vi "Read status lines.vi"(11 "httpResponse in":refnum<class "httpResponse.lvclass">) -> (1 "status chain":string[](array[string]), 2 "status":string, 3 "httpResponse out":refnum<class "httpResponse.lvclass">)   [LabVIEW 2020, in "httpClient.lvlib" / "httpResponse.lvclass"]
uses:
  httpResponse.lvclass
  httpResponse.lvclass/httpResponse.ctl
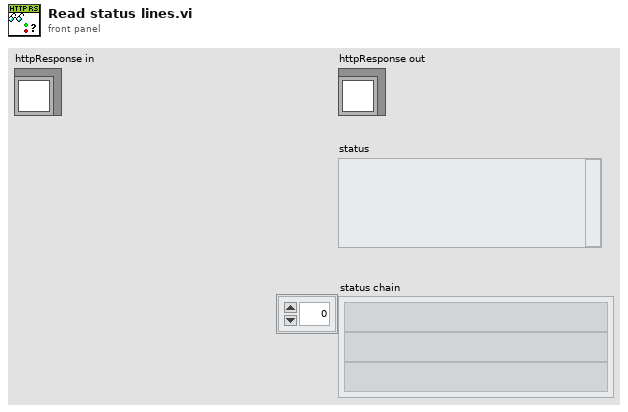
[diagram p1: front panel]
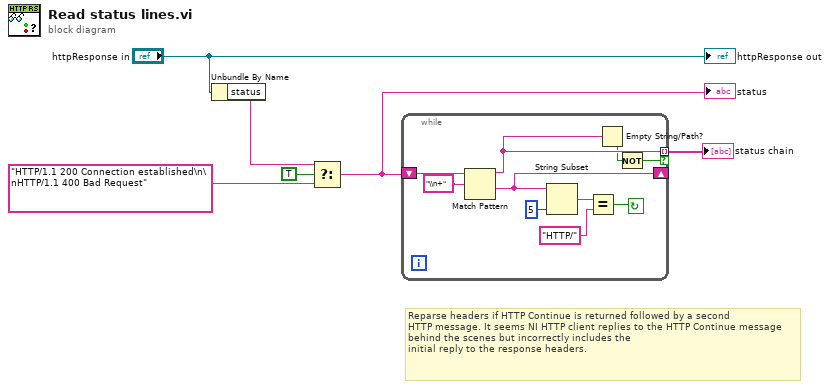
[diagram p0: block diagram]
diagram:
  # "Reparse headers if HTTP Continue is returned followed by a second\nHTTP message. It seems NI HTTP client replies to the HTTP Continue message behind the scenes but incorrectly includes the\ninitial reply to the response headers."
  n1 = Unbundle By Name("httpResponse in") -> ("status"=w2:string)
  n2 = Select(t=w2, s=TRUE, f="HTTP/1.1 200 Connection established\n\nHTTP/1.1 400 Bad Request" ("regular expression")) -> (s? t:f=w1:string)
  "status" <- w1
  n3 = while {
    shift-right: [w12] -> _
    shift-left: w1 -> [w16]
    tunnel: [w9] -> w3 mode=indexing if=w7
    stop <- w10 continue-if-true
    n4 = Match Pattern(string=w16, regular expression="\\n+") -> (before substring=w9:string, after substring=w12:string)  [unwired: 1 in, 2 out]
    n5 = String Subset(string=w12, length (rest)=5 ("length (rest)")) -> (substring=w13:string)  [unwired: 1 in]
    n6 = Equal?(x=w13, y="HTTP/") -> (x = y?=w10:bool)
    n7 = Empty String/Path?(string/path=w9) -> (empty?=w8:bool)
    n8 = Not(x=w8) -> (.not. x?=w7:bool)
  }
  "status chain" <- w3
  "httpResponse out" <- "httpResponse in"
